vi "Create Image Constructor Class.vi"(8 "error in (no error)":errorcluster, 11 "Channel in":refnum<class "Channel.lvclass">) -> (0 "error out":errorcluster, 3 "Channel out":refnum<class "Channel.lvclass">)   [LabVIEW 2018, in "Channel.lvclass"]
uses:
  Channel.lvclass
  Simulated_Image_Constructor/Simulated_Image_Constructor.lvclass
  Simulated_Header/Simulated_Header.lvclass
  Image Constructor/Image Constructor.lvclass
  C:/Users/observer/Desktop/SPARC4_ACS/SPARC4_ACS/Simulated_Image_Constructor/Simulated_Image_Constructor.lvclass
  CCDCamera/CCDCamera.lvclass
  C:/Users/observer/Desktop/SPARC4_ACS/SPARC4_ACS/Simulated_CCD_Camera/Simulated_CCD_Camera.lvclass
  Cooler/Cooler.lvclass
  C:/Users/observer/Desktop/SPARC4_ACS/SPARC4_ACS/Simulated_Cooler/Simulated_Cooler.lvclass
  Header/Header.lvclass
  C:/Users/observer/Desktop/SPARC4_ACS/SPARC4_ACS/Simulated_Header/Simulated_Header.lvclass
  Simulated_Image_Constructor/Simulated_Image_Constructor.lvclass/Simulated_Image_Constructor.ctl
  Channel.lvclass/Channel.ctl
  Save Image/Save Image.lvclass
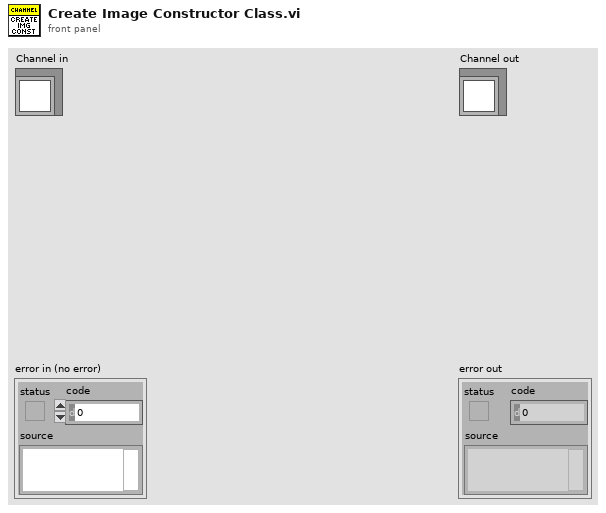
[diagram p1: front panel]
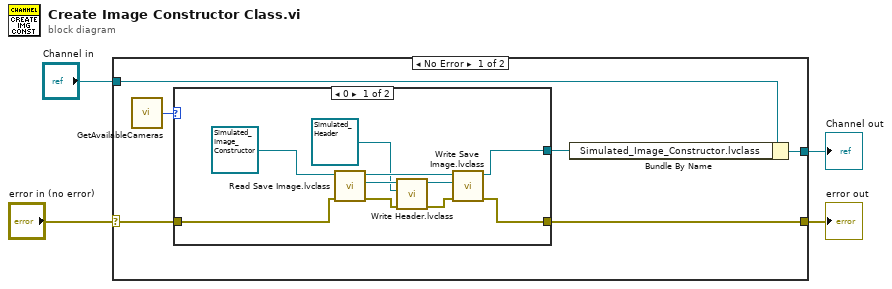
[diagram p0: block diagram]
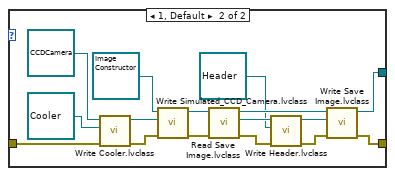
[diagram p2: hidden frame]
diagram:
  n1 = case shown="No Error" "error in (no error)" {
    selector: "error in (no error)" -> [w7 w38]
    tunnel: [w5 w38] -> w3
    tunnel: [w10 w37] -> w1
    tunnel: "Channel in" -> [w9 w37]
    frame No Error {
      n2 = call <userlib>:"GetAvailableCameras.vi"() -> ("totalCameras"=w8:i32)  [unwired: 3 in, 2 out]
      n3 = case shown="0" w8 {
        tunnel: w7 -> [w18 w33]
        tunnel: [w12 w22] -> w6
        tunnel: [w13 w21] -> w5
        frame 0 {
          n4 = call "Read Save Image.lvclass.vi"("error in (no error)"=w18, "Image Constructor in"=refnum<class "Simulated_Image_Constructor.lvclass"> refnum ("Simulated_Image_Constructor.lvclass")) -> ("error out"=w17:errorcluster, "Save Image.lvclass"=w16:refnum<class "Save Image.lvclass">, "Image Constructor out"=w20:refnum<class "Simulated_Image_Constructor.lvclass">)  [unwired: 7 in]
          n5 = call "Write Header.lvclass.vi"("error in (no error)"=w17, "Simulated_Header.lvclass"=refnum<class "Simulated_Header.lvclass"> refnum, "Save Image in"=w16) -> ("error out"=w14:errorcluster, "Save Image out"=w15:refnum<class "Save Image.lvclass">)  [unwired: 7 in]
          n6 = call "Write Save Image.lvclass.vi"("error in (no error)"=w14, "Save Image.lvclass"=w15, "Image Constructor in"=w20) -> ("error out"=w13:errorcluster, "Image Constructor out"=w12:refnum<class "Simulated_Image_Constructor.lvclass">)  [unwired: 7 in]
        }
        frame 1, Default {
          n7 = call-dynamic "Write Cooler.lvclass.vi"("error in (no error)"=w33, "Simulated_Cooler.lvclass"=refnum<class "Cooler.lvclass"> refnum ("Cooler.lvclass"), "CCDCamera in"=refnum<class "CCDCamera.lvclass"> refnum ("CCDCamera.lvclass")) -> ("error out"=w31:errorcluster, "CCDCamera out"=w32:refnum<class "CCDCamera.lvclass">)  [unwired: 7 in]
          n8 = call "Write Simulated_CCD_Camera.lvclass.vi"("error in (no error)"=w31, "Simulated_CCD_Camera.lvclass"=w32, "Image Constructor in"=refnum<class "Image Constructor.lvclass"> refnum ("Image Constructor.lvclass")) -> ("error out"=w29:errorcluster, "Image Constructor out"=w30:refnum<class "Image Constructor.lvclass">)  [unwired: 7 in]
          n9 = call "Read Save Image.lvclass.vi"("error in (no error)"=w29, "Image Constructor in"=w30) -> ("error out"=w25:errorcluster, "Save Image.lvclass"=w27:refnum<class "Save Image.lvclass">, "Image Constructor out"=w28:refnum<class "Image Constructor.lvclass">)  [unwired: 7 in]
          n10 = call "Write Header.lvclass.vi"("error in (no error)"=w25, "Simulated_Header.lvclass"=refnum<class "Header.lvclass"> refnum ("Header.lvclass"), "Save Image in"=w27) -> ("error out"=w24:errorcluster, "Save Image out"=w26:refnum<class "Save Image.lvclass">)  [unwired: 7 in]
          n11 = call "Write Save Image.lvclass.vi"("error in (no error)"=w24, "Save Image.lvclass"=w26, "Image Constructor in"=w28) -> ("error out"=w21:errorcluster, "Image Constructor out"=w22:refnum<class "Image Constructor.lvclass">)  [unwired: 7 in]
        }
      }
      n12 = Bundle By Name(cluster=w9, "Simulated_Image_Constructor.lvclass"=w6) -> (w10:refnum<class "Channel.lvclass">)
    }
    frame Error {
    }
  }
  "error out" <- w3
  "Channel out" <- w1
